vi "phan_upgrade9_12.vi"() -> ()   [LabVIEW 2019]
uses:
  <vilib>/myRIO/Instrument Drivers/Onboard IO/I2C/typedefs/I2C User Configuration.ctl
  <vilib>/myRIO/Instrument Drivers/Onboard IO/I2C/typedefs/I2C Transfer Rate.ctl
  <vilib>/Platform/TimedLoop/XDataNode/timing_clust.ctl
  <vilib>/Platform/TimedLoop/XDataNode/nitl_modes.ctl
  <vilib>/Platform/TimedLoop/XDataNode/wakeup.ctl
  <vilib>/myRIO/Instrument Drivers/Onboard IO/I2C/typedefs/I2C Reference.ctl
  <vilib>/myRIO/Common/Instrument Driver Framework/Utilities/typedefs/myRIO Generic Hardware Reference.ctl
  <vilib>/myRIO/Common/Instrument Driver Framework/Utilities/typedefs/Hardware Version Enum.ctl
  <vilib>/myRIO/Common/Instrument Driver Framework/Utilities/typedefs/myRIO v1.0 Reference.ctl
  <vilib>/myRIO/Common/Instrument Driver Framework/Utilities/typedefs/Generic FPGA Reference.ctl
  <vilib>/myRIO/Common/Instrument Driver Framework/myRIO v1.0/I2C/typedefs/I2C Channels Enum.ctl
  <vilib>/myRIO/Instrument Drivers/Onboard IO/I2C/typedefs/I2C Configuration.ctl
  <vilib>/userDefined/High Color/nirio_resource_hc.ctl
  <vilib>/myRIO/Common/Instrument Driver Framework/myRIO v1.0/I2C/vis/myRIO v1.1 Open I2C.vi
  <vilib>/myRIO/Common/Instrument Driver Framework/Utilities/vis/Validate Channels.vi
  <vilib>/myRIO/Common/Instrument Driver Framework/myRIO v1.0/I2C/vis/myRIO v1.0 Reserve I2C.vi
  <vilib>/myRIO/Common/Instrument Driver Framework/myRIO v1.0/UART/vis/myRIO v1.0 Close UART.vi
  <vilib>/myRIO/Common/Instrument Driver Framework/myRIO v1.0/I2C/vis/myRIO v1.0 Build MUX Configuration I2C.vi
  <vilib>/myRIO/Common/Instrument Driver Framework/myRIO v1.0/Resource Manager/vis/myRIO v1.0 Reserve Channel List.vi
  <vilib>/myRIO/Common/Instrument Driver Framework/myRIO v1.0/Resource Manager/vis/myRIO v1.0 Create Configuration List.vi
  <vilib>/myRIO/Common/Instrument Driver Framework/myRIO v1.0/Resource Manager/vis/myRIO v1.0 Reserve Channel.vi
  <vilib>/myRIO/Common/Instrument Driver Framework/myRIO v1.0/Resource Manager/vis/myRIO v1.0 Unreserve Channel.vi
  <vilib>/myRIO/Common/Instrument Driver Framework/myRIO v1.0/Resource Manager/vis/myRIO v1.0 Build Mutex Name.vi
  <vilib>/Utility/VariantDataType/GetNumericInfo.vi
  <vilib>/Utility/error.llb/Error Cluster From Error Code.vi
  <vilib>/myRIO/Common/Instrument Driver Framework/myRIO v1.0/myRIO v1.1 Open.vi
  <vilib>/myRIO/Common/Instrument Driver Framework/Utilities/vis/IO Manager.vi
  <vilib>/myRIO/Common/Instrument Driver Framework/Utilities/vis/Configuration Manager.vi
  <vilib>/myRIO/Common/Instrument Driver Framework/myRIO v1.0/Resource Manager/vis/myRIO v1.0 Configure IO.vi
  <vilib>/myRIO/Common/Instrument Driver Framework/myRIO v1.0/myRIO v1.0 Close.vi
  <vilib>/myRIO/Common/Instrument Driver Framework/myRIO v1.0/I2C/vis/myRIO v1.0 Configure I2C.vi
  <vilib>/myRIO/Common/Instrument Driver Framework/myRIO v1.0/I2C/vis/myRIO v1.0 Write I2C.vi
  <vilib>/myRIO/Common/Instrument Driver Framework/myRIO v1.0/I2C/vis/myRIO v1.0 Read I2C.vi
  <vilib>/myRIO/Common/Instrument Driver Framework/Utilities/vis/FPGA Ref Manager.vi
  <vilib>/myRIO/Common/Instrument Driver Framework/myRIO v1.0/myRIO v1.0 Reset FPGA.vi
  <vilib>/myRIO/Common/Instrument Driver Framework/myRIO v1.0/IRQ/vis/myRIO v1.0 IRQ Info FGV.vi
  <vilib>/myRIO/Common/Instrument Driver Framework/myRIO v1.0/IRQ/vis/myRIO v1.0 Timer IRQ Info FGV.vi
  <vilib>/myRIO/Common/Instrument Driver Framework/myRIO v1.0/IRQ/vis/myRIO v1.0 ISR Agent.vi
  <vilib>/myRIO/Instrument Drivers/Utilities/vis/Reset Index.vi
  <vilib>/myRIO/Common/Instrument Driver Framework/myRIO v1.0/Resource Manager/vis/myRIO v1.0 Block Write Resource Manager.vi
  <vilib>/platform/TimedLoop/XDataNode/XDataNode.xnode
  <vilib>/myRIO/Instrument Drivers/Onboard IO/I2C/vis/myRIO I2C Open.xnode
  <vilib>/Platform/TimedLoop/XDataNode/XDNodeRunTimeDep.lvlib
  <vilib>/ptbypt/NI_PtbyPt.lvlib
  <vilib>/myRIO/Instrument Drivers/Onboard IO/I2C/I2C.lvlib
  <vilib>/myRIO/Instrument Drivers/Utilities/Utilities.lvlib
panel:
  out "y":dbl(graph)
  out "x":dbl(graph)
  out "theta_ph":dbl
  out "offset":dbl
  out "gocphanhoi":dbl
  out "y_1":dbl
  out "x_1":dbl
  out "y_0":dbl
  out "x_0":dbl
  out "wpre":dbl
  out "yo":dbl
  out "xo":dbl
  out "phi_ph":dbl
  out "wdk":dbl
  out "phi_sp":dbl
  in  "Kiw":dbl
  in  "Kpw":dbl=3.0
  in  "Kdw":dbl
  out "Vxdk":dbl
  out "Vydk":dbl
  in  "Kdv3":dbl
  in  "Kiv3":dbl=30.0
  in  "Kpv3":dbl=0.7
  in  "Kdv2":dbl
  in  "Kiv2":dbl=30.0
  in  "Kpv2":dbl=0.7
  out "Ts":dbl=10.0
  out "sailechvitri":cluster{"e_phi":dbl, "e_x":dbl, "e_y":dbl}(graph)
  in  "Kdxy":dbl
  in  "Kixy":dbl
  in  "Kpxy":dbl=4.0
  in  "?":T1(tab)
  out "time":dbl
  in  "phi_start":dbl=1.57 format="%#_13g"
  in  "phi_end":dbl=18.85
  in  "x0":dbl
  in  "w":dbl=0.2
  in  "y0":dbl
  in  "R":dbl=1.0
  in  "R":dbl=0.6
  in  "phi_end":dbl=18.85
  in  "phi_start":dbl format="%#_13g"
  in  "x0":dbl
  in  "w":dbl=0.5
  out "time 2":dbl
  in  "y0":dbl
  out "time":dbl
  in  "x":dbl
  in  "y":dbl
  in  "CONT":bool
  in  "vantoc":dbl=0.3
  in  "x0":dbl
  in  "y0":dbl
  in  "vx":dbl
  in  "vy":dbl
  out "time":dbl
  out "time 3":dbl
  in  "phi_start 2":dbl format="%#_13g"
  in  "phi_end 2":dbl=31.4
  in  "x0 2":dbl
  in  "w 2":dbl=0.2
  in  "y0 2":dbl
  out "w_ph3":dbl
  out "w_ph2":dbl
  out "w_ph1":dbl
  in  "RESETMAP":bool=TRUE caption="Reset"
  out "duty3":dbl
  out "duty2":dbl
  out "duty1":dbl
  in  "RESET":bool
  out "Y_sp":dbl
  out "X_sp":dbl
  out "Y_ph":dbl
  out "X_ph":dbl
  out "Map":cluster{"Y":dbl[], "Y":dbl[]}[](graph)
  out "V3_sp":dbl
  out "V3_ph":dbl
  out "VAN TOC":T2(graph)
  in  "Kdv1":dbl
  in  "Kiv1":dbl=30.0
  in  "Kpv1":dbl=0.7
  out "V2_ph":dbl
  out "V1_ph":dbl
  out "V2_sp":dbl
  out "V1_sp":dbl
  in  "START":bool
  # "HE THONG"
  # "PID VI TRI"
  # "PID TOC DO"
  # "VI TRI DIEU KHIEN\n(m)"
  # "VI TRI PHAN HOI\n(m)"
  # "Van toc dat"
  # "VAN TOC DIEU KHIEN\n(m/s)"
  # "VAN TOC PHAN HOI\n(m/s)"
  # "DUTY"
  # "TOC DO PHAN HOI (rad/s)"
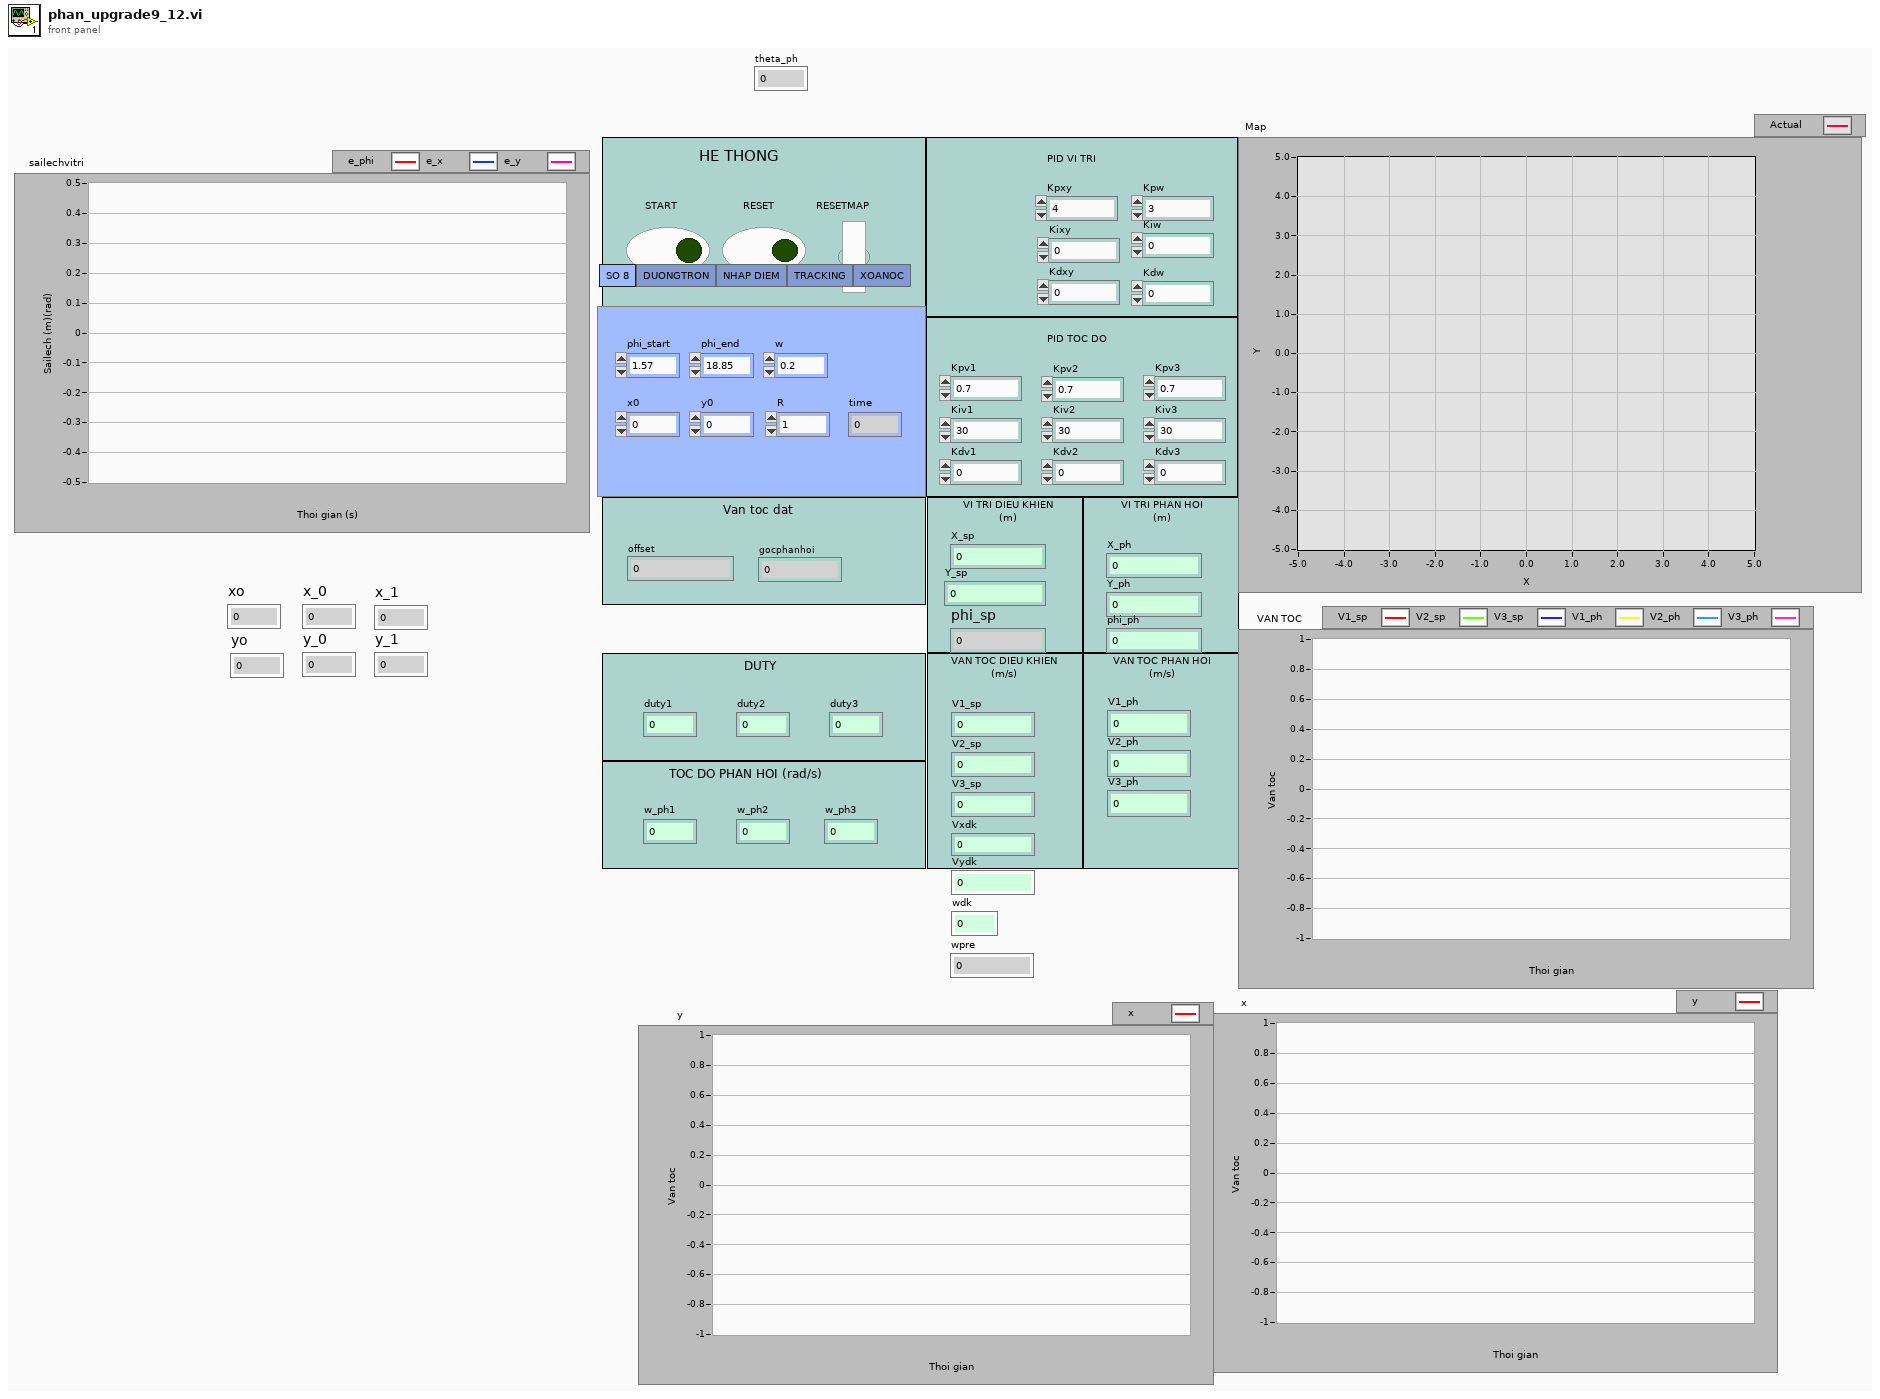
[diagram p1: front panel]
types:
  T1 = enum32{"SO 8", "DUONGTRON", "NHAP DIEM", "TRACKING", "XOANOC"}
  T2 = cluster{dbl, dbl, "V1_ph":dbl, "V2_ph":dbl, dbl, "V3_ph":dbl}
  T3 = typedef "I2C.lvlib/I2C User Configuration.ctl" = cluster{"I2C Transfer Rate":T4}
  T4 = typedef "I2C.lvlib/I2C Transfer Rate.ctl" = enum16{"Standard mode (100 kbps)", "Fast mode (400 kbps)"}
  T5 = typedef "XDNodeRunTimeDep.lvlib/timing_clust.ctl" = cluster{"Expected End [f-1]":u64, "Actual End [f-1]":u64, "Finished Late? [f-1]":bool, "Expected End [i-1]":u64, "Actual End [i-1]":u64, "Finished Late? [i-1]":bool, "Expected Start [i]":u64, "Actual Start [i]":u64, "Expected Start [f]":u64, "Actual Start [f]":u64, "Source Name":string, "Structure Name":string, "Period":i64, "Deadline":i64, "Offset":i64, "Start":i64, "Priority":i32, "Timeout":i32, "Mode":T6, "Wakeup Reason":T7, "Error":errorcluster, "Source Type":string, "Secondary Source Type":string, "Global End Time":u64, "Global Start Time":u64, "Frame Duration":u64, "Iteration Duration":u64, "Assigned CPU":i32, "I/O Scan Engine Mode":u32}
  T6 = typedef "XDNodeRunTimeDep.lvlib/nitl_modes.ctl" = enum32{"No Change", "Process missed periods, maintain original phase", "Discard missed periods, maintain original phase", "Process missed periods, ignore original phase", "Discard missed periods, ignore original phase"}
  T7 = typedef "XDNodeRunTimeDep.lvlib/wakeup.ctl" = enum32{"Normal", "Aborted", "Asynchronous wakeup", "Timing source error", "Timed loop error", "Timeout"}
  T8 = typedef "I2C.lvlib/I2C Reference.ctl" = cluster{"myRIO Reference":T9, "I2C Channels Enum":T13, "I2C Configuration":T14}
  T9 = typedef "myRIO Generic Hardware Reference.ctl" = cluster{"myRIO Model":T10, "myRIO Hardware Reference":T11}
  T10 = typedef "Hardware Version Enum.ctl" = enum16{"Unknown", "myRIO-1900", "myRIO-1950", "roboRIO", "NI ELVIS RIO CM", "ELVIS III"}
  T11 = typedef "myRIO v1.0 Reference.ctl" = cluster{"Generic FPGA Reference":T12, "Allow multiple opens":bool}
  T12 = typedef "Generic FPGA Reference.ctl" = refnum<k20>
  T13 = typedef "I2C Channels Enum.ctl" = enum16{"Not Connected", "A/I2C", "B/I2C", "I2C/I2C"}
  T14 = typedef "I2C.lvlib/I2C Configuration.ctl" = cluster{"I2C Transfer Rate":T4}
  T15 = cluster{"V1_sp":dbl, "V2_sp":dbl, "V3_sp":dbl, "V_ph1":dbl, "V_ph2":dbl, "V_ph3":dbl}
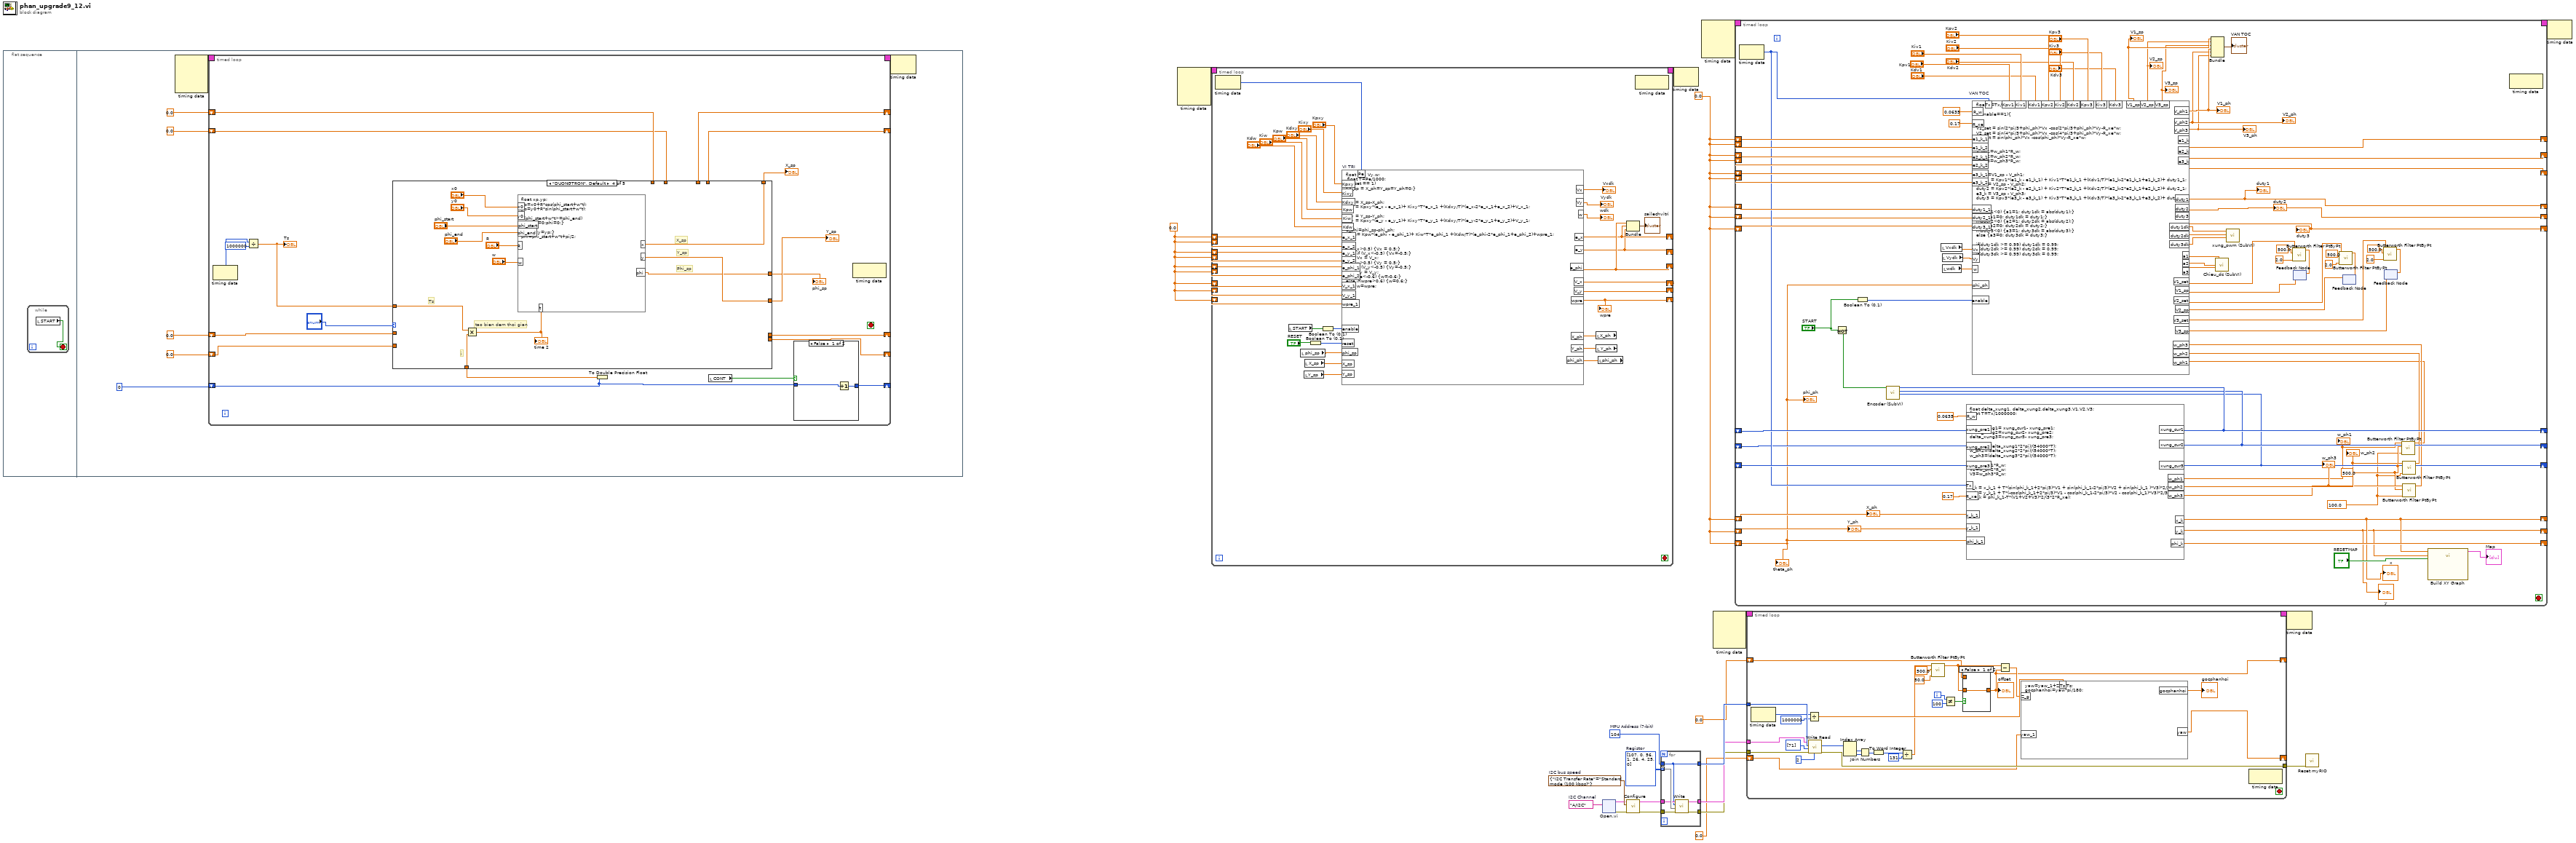
[diagram p0: block diagram]
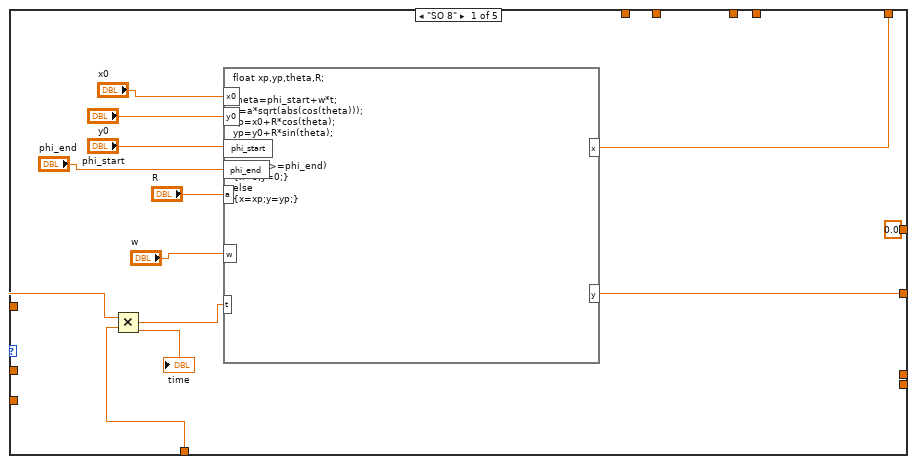
[diagram p3: hidden frame]
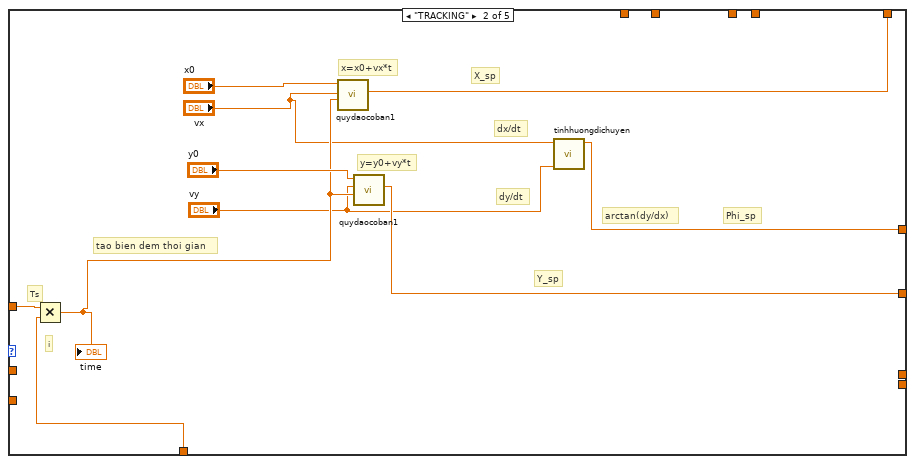
[diagram p4: hidden frame]
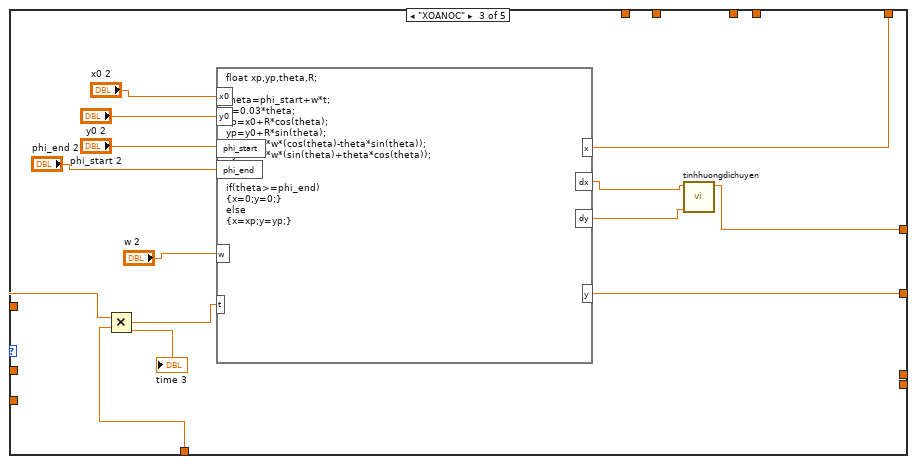
[diagram p5: hidden frame]
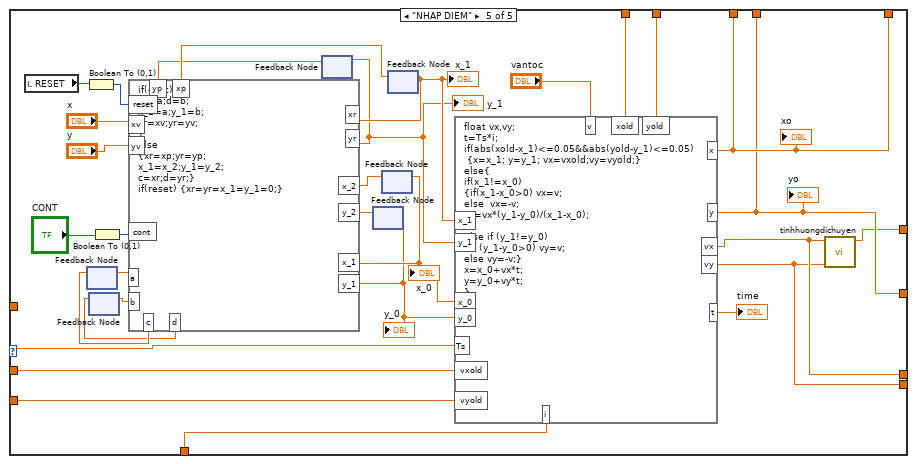
[diagram p6: hidden frame]
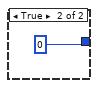
[diagram p7: hidden frame]
diagram:
  w9 = u8[][] [[107, 0], [56, 1], [26, 4], [25, 0]]  # Registor
  w8 = u8 104  # MPU Address (7-bit)
  w13 = T3 {"I2C Transfer Rate"=enum."Standard mode (100 kbps)"}  # I2C bus speed
  w14 = tag "A/I2C"  # I2C Channel
  w17 = 0.0 ("e_x")
  w18 = 0.0 ("e1")
  n1 = flat-sequence {
    frame #0 {
      n2 = while {
        stop <- w23 stop-if-true
        n3 = local read "START"() -> (w23:bool)
      }
    }
    frame #1 {
      n4 = node-c288() -> (w30:T5)  [unwired: 4 in]
      n5 = timed-loop {
        timing: w30 -> [_]
        timing-out: [_] -> w29
        shift-right: [w48] -> _
        shift-left: 0 -> [w47]
        shift-right: [w38] -> _
        shift-left: 0.0 -> [w36]
        shift-right: [w37] -> _
        shift-left: 0.0 -> [w35]
        shift-right: [w34] -> _
        shift-left: 0.0 ("x") -> [w32]
        shift-right: [w33] -> _
        shift-left: 0.0 ("y") -> [w31]
        stop <- _ stop-if-true
        n6 = node-c288() -> (w46:i64)  [unwired: 1 in]
        n7 = Divide(x=w46, y=i64 1000000) -> (x/y=w43:dbl)
        "Ts" <- w43
        n8 = To Double Precision Float(number=w47) -> (double precision float=w49:dbl)
        n9 = case shown="\"DUONGTRON\", Default" "?" {
          tunnel: w49 -> [w60 w71 w77 w95 w127]
          tunnel: [w52 w68 w75 w87 w101] -> w42
          tunnel: [w51 w65 w76 w86 w100] -> w41
          tunnel: [0.0 ("phi_0") w62 w72 w85 w97] -> w40
          tunnel: w43 -> [w61 w70 w78 w96 w107]
          tunnel: [_ _ _ _ w105] -> w38
          tunnel: [_ _ _ _ w104] -> w37
          tunnel: w36 -> [_ _ _ _ w103]
          tunnel: w35 -> [_ _ _ _ w102]
          tunnel: [_ _ _ _ w101] -> w34
          tunnel: [_ _ _ _ w100] -> w33
          tunnel: w32 -> [_ _ _ _ w99]
          tunnel: w31 -> [_ _ _ _ w98]
          frame "SO 8" {
            n10 = Multiply(x=w61, y=w60) -> (x*y=w59:dbl)
            "time" <- w59
            n11 = formula code="float xp,yp,theta,R;\n\ntheta=phi_start+w*t;\nR=a*sqrt(abs(cos(theta)));\nxp=x0+R*cos(theta);\nyp=y0+R*sin(theta);\n\n\nif(theta>=phi_end)\n{x=0;y=0;}\nelse\n{x=xp;y=yp;}"("t"=w59, "w"="w", "x0"="x0", "y0"="y0", "phi_start"="phi_start", "phi_end"="phi_end", "a"="R") -> ("x"=w52:dbl, "y"=w51:dbl)
          }
          frame "TRACKING" {
            # "Y_sp"
            # "Phi_sp"
            # "X_sp"
            # "arctan(dy/dx)"
            # "dy/dt"
            # "dx/dt"
            # "Ts"
            # "i"
            # "y=y0+vy*t"
            # "x=x0+vx*t"
            # "tao bien dem thoi gian"
            n12 = Multiply(x=w70, y=w71) -> (x*y=w66:dbl)
            "time" <- w66
            n13 = call "quydaocoban1.vi"("t"=w66, "v"="vx", "S0"="x0") -> ("S"=w68:dbl)  [unwired: 8 in]
            n14 = call "quydaocoban1.vi"("t"=w66, "v"="vy", "S0"="y0") -> ("S"=w65:dbl)  [unwired: 8 in]
            n15 = call "tinhhuongdichuyen.vi"("dy"="vy", "dx"="vx") -> ("phi"=w62:dbl)  [unwired: 9 in]
          }
          frame "XOANOC" {
            n16 = Multiply(x=w78, y=w77) -> (x*y=w84:dbl)
            "time 3" <- w84
            n17 = formula code="float xp,yp,theta,R;\n\ntheta=phi_start+w*t;\nR=0.03*theta;\nxp=x0+R*cos(theta);\nyp=y0+R*sin(theta);\ndx=0.03*w*(cos(theta)-theta*sin(theta));\ndy=0.03*w*(sin(theta)+theta*cos(theta));\n\n\nif(theta>=phi_end)\n{x=0;y=0;}\nelse\n{x=xp;y=yp;}"("t"=w84, "w"="w 2", "x0"="x0 2", "y0"="y0 2", "phi_start"="phi_start 2", "phi_end"="phi_end 2") -> ("x"=w75:dbl, "y"=w76:dbl, "dx"=w74:dbl, "dy"=w73:dbl)
            n18 = call "tinhhuongdichuyen.vi"("dy"=w73, "dx"=w74) -> ("phi"=w72:dbl)  [unwired: 9 in]
          }
          frame "DUONGTRON", Default {
            # "Phi_sp"
            # "Y_sp"
            # "X_sp"
            # "i"
            # "Ts"
            # "tao bien dem thoi gian"
            n19 = Multiply(x=w96, y=w95) -> (x*y=w94:dbl)
            "time 2" <- w94
            n20 = formula code="float xp,yp;\nxp=x0+R*cos(phi_start+w*t);\nyp=y0+R*sin(phi_start+w*t);\n\nif(phi_start+w*t>=phi_end)\n{x=0;y=0;phi=0;}\nelse\n{x=xp;y=yp;}\nphi=phi_start+w*t+pi/2;"("t"=w94, "w"="w", "x0"="x0", "y0"="y0", "phi_start"="phi_start", "phi_end"="phi_end", "R"="R") -> ("x"=w87:dbl, "y"=w86:dbl, "phi"=w85:dbl)
          }
          frame "NHAP DIEM" {
            n21 = local read "RESET"() -> (w109:bool)
            n22 = Boolean To (0,1)(Boolean=w109) -> (0, 1=w108:i16)
            n23 = feedback #1() -> (w112:dbl)  [unwired: 1 in]
            n24 = feedback #2() -> (w110:dbl)  [unwired: 1 in]
            n25 = Boolean To (0,1)(Boolean="CONT") -> (0, 1=w124:i16)
            n26 = feedback #3() -> (w118:dbl)  [unwired: 1 in]
            n27 = feedback #4() -> (w115:dbl)  [unwired: 1 in]
            n28 = feedback #5() -> (w117:dbl)  [unwired: 1 in]
            n29 = feedback #6() -> (w119:dbl)  [unwired: 1 in]
            n30 = formula code="if(cont)\n{c=a;d=b;\nx_1=a;y_1=b;\nxr=xv;yr=yv;\n}\nelse \n{xr=xp;yr=yp;\nx_1=x_2;y_1=y_2;\nc=xr;d=yr;}\nif(reset) {xr=yr=x_1=y_1=0;}"("cont"=w124, "xv"="x", "yv"="y", "yp"=w118, "xp"=w119, "x_2"=w117, "y_2"=w115, "a"=w112, "b"=w110, "reset"=w108) -> ("xr"=w121:dbl, "yr"=w120:dbl, "x_1"=w116:dbl, "y_1"=w114:dbl, "c"=w113:dbl, "d"=w111:dbl)
            "x_0" <- w116
            "y_0" <- w114
            "x_1" <- w121
            "y_1" <- w120
            n31 = feedback-in #1(w113) -> ()
            n32 = feedback-in #2(w111) -> ()
            n33 = feedback-in #3(w120) -> ()
            n34 = feedback-in #4(w114) -> ()
            n35 = feedback-in #5(w116) -> ()
            n36 = feedback-in #6(w121) -> ()
            n37 = formula code="float vx,vy;\nt=Ts*i;\nif(abs(xold-x_1)<=0.05&&abs(yold-y_1)<=0.05)\n {x=x_1; y=y_1; vx=vxold;vy=vyold;}\nelse{\nif(x_1!=x_0)\n{if(x_1-x_0>0) vx=v;\nelse  vx=-v;\nvy=vx*(y_1-y_0)/(x_1-x_0);\n}\nelse if (y_1!=y_0) \n{if (y_1-y_0>0) vy=v;\nelse vy=-v;}\nx=x_0+vx*t;\ny=y_0+vy*t;\n}"("i"=w127, "x_1"=w121, "y_1"=w120, "x_0"=w116, "y_0"=w114, "Ts"=w107, "v"="vantoc", "xold"=w99, "yold"=w98, "vxold"=w103, "vyold"=w102) -> ("x"=w101:dbl, "y"=w100:dbl, "vx"=w105:dbl, "t"=→"time":dbl, "vy"=w104:dbl)
            "xo" <- w101
            "yo" <- w100
            n38 = call "tinhhuongdichuyen.vi"("dy"=w104, "dx"=w105) -> ("phi"=w97:dbl)  [unwired: 9 in]
          }
        }
        "X_sp" <- w42
        "Y_sp" <- w41
        "phi_sp" <- w40
        n39 = local read "CONT"() -> (w44:bool)
        n40 = case shown="False" w44 {
          tunnel: [w129 0] -> w48
          tunnel: w47 -> [w128 _]
          frame False {
            n41 = Increment(x=w128) -> (x+1=w129:i32)
          }
          frame True {
          }
        }
        n42 = node-c288() -> ()  [unwired: 1 in, 1 out]
      }
      n43 = node-c288(w29) -> ()  [unwired: 1 out]
    }
  }
  n44 = node-c288() -> (w20:T5)  [unwired: 4 in]
  n45 = timed-loop {
    timing: w20 -> [_]
    timing-out: [_] -> w19
    shift-right: [w156] -> _
    shift-left: w17 -> [w164]
    shift-left: w17 -> [w163]
    shift-right: [w142] -> _
    shift-left: w17 -> [w162]
    shift-left: w17 -> [w161]
    shift-right: [w157] -> _
    shift-left: w17 -> [w160]
    shift-left: w17 -> [w159]
    shift-right: [w147] -> _
    shift-left: w17 -> [w150]
    shift-right: [w146] -> _
    shift-left: w17 -> [w149]
    shift-right: [w145] -> _
    shift-left: w17 -> [w148]
    stop <- _ stop-if-true
    # "Gioihantocdo"
    # "BodieukhienPIDvitri"
    n46 = node-c288() -> (w171:i64)  [unwired: 1 in]
    n47 = local read "START"() -> (w144:bool)
    n48 = local read "phi_sp"() -> (w140:dbl)
    n49 = local read "Y_sp"() -> (w139:dbl)
    n50 = local read "X_sp"() -> (w141:dbl)
    n51 = Boolean To (0,1)(Boolean="RESET") -> (0, 1=w154:i16)
    n52 = Boolean To (0,1)(Boolean=w144) -> (0, 1=w143:i16)
    n53 = local read "X_ph"() -> (w153:dbl)
    n54 = local read "Y_ph"() -> (w152:dbl)
    n55 = local read "phi_ph"() -> (w151:dbl)
    n56 = formula code="float  Vx, Vy,w;\n float T=Pe/1000;\nif(reset == 1)\n{X_sp = X_ph=Y_sp=Y_ph=0;}\n \n\ne_x = X_sp-X_ph; \nV_x = Kpxy*(e_x - e_x_1)+ Kixy*T*e_x_1 +(Kdxy/T)*(e_x-2*e_x_1+e_x_2)+V_x_1;\n\ne_y = Y_sp-Y_ph; \nV_y = Kpxy*(e_y - e_y_1)+ Kixy*T*e_y_1 +(Kdxy/T)*(e_y-2*e_y_1+e_y_2)+V_y_1;\n\ne_phi=phi_sp-phi_ph;\nwpre= Kpw*(e_phi - e_phi_1)+ Kiw*T*e_phi_1 +(Kdw/T)*(e_phi-2*e_phi_1+e_phi_2)+wpre_1;\n\n\nif (V_x>0.5) {Vx = 0.5;} \nelse if (V_x<-0.5) {Vx=-0.5;}\nelse Vx = V_x;\nif (V_y>0.5) {Vy = 0.5;} \nelse if (V_y<-0.5) {Vy=-0.5;}\nelse Vy = V_y;\nif (wpre<-0.6) {w=-0.6;}\nelse if(wpre>0.6) {w=0.6;}\nelse w=wpre;" "VI TRI"("Kpxy"="Kpxy", "Kixy"="Kixy", "Kdxy"="Kdxy", "Kpw"="Kpw", "Kiw"="Kiw", "Kdw"="Kdw", "Pe"=w171, "e_x_1"=w164, "e_x_2"=w163, "e_y_1"=w162, "e_y_2"=w161, "e_phi_1"=w160, "e_phi_2"=w159, "reset"=w154, "phi_sp"=w140, "X_sp"=w141, "Y_sp"=w139, "X_ph"=w153, "Y_ph"=w152, "phi_ph"=w151, "V_x_1"=w150, "V_y_1"=w149, "wpre_1"=w148, "enable"=w143) -> ("e_x"=w156:dbl, "e_y"=w142:dbl, "e_phi"=w157:dbl, "Vx"=→"Vxdk":dbl, "Vy"=→"Vydk":dbl, "w"=→"wdk":dbl, "V_x"=w147:dbl, "V_y"=w146:dbl, "wpre"=w145:dbl)
    "wpre" <- w145
    n57 = Bundle("e_phi"=w157, "e_x"=w156, "e_y"=w142) -> (→"sailechvitri":cluster{"e_phi":dbl, "e_x":dbl, "e_y":dbl})  [unwired: 1 in]
    n58 = node-c288() -> ()  [unwired: 1 in, 1 out]
  }
  n59 = xnode "Open.vi"("Channel Name"=w14) -> ("error out"=w11:errorcluster, "I2C Ref Out"=w12:T8)  [unwired: 2 in]
  n60 = call <vilib>:"Configure.vi"("error in (no error)"=w11, "I2C User Configuration"=w13, "I2C Ref In"=w12) -> ("error out"=w10:errorcluster, "I2C Ref Out"=w6:T8)  [unwired: 7 in]
  n61 = for {
    tunnel: w10 -> [w180]
    tunnel: w8 -> [w177]
    tunnel: w9 -> [w179] mode=indexing
    tunnel: w6 -> [w178]
    tunnel: [w177] -> w5
    tunnel: [w176] -> w4
    tunnel: [w175] -> w3
    n62 = call <vilib>:"Write.vi"("error in (no error)"=w180, "Bytes to Write"=w179, "Slave Address (7-bit)"=w177, "I2C Ref In"=w178) -> ("error out"=w175:errorcluster, "I2C Ref Out"=w176:T8)  [unwired: 6 in]
  }
  n63 = node-c288(w19) -> ()  [unwired: 1 out]
  n64 = node-c288() -> (w22:T5)  [unwired: 4 in]
  n65 = node-c288() -> (w16:T5)  [unwired: 4 in]
  n66 = timed-loop {
    timing: w22 -> [_]
    timing-out: [_] -> w21
    shift-right: [w265] -> _
    shift-left: w18 -> [w263]
    shift-right: [w264] -> _
    shift-left: w18 -> [w242]
    shift-right: [w257] -> _
    shift-left: w18 -> [w256]
    shift-right: [w182] -> _
    shift-left: w18 -> [w200]
    shift-right: [w181] -> _
    shift-left: w18 -> [w199]
    shift-right: [w253] -> _
    shift-left: w18 -> [w251]
    shift-right: [w252] -> _
    shift-left: w18 -> [w201]
    shift-right: [w207] -> _
    shift-left: w18 -> [w250]
    shift-right: [w245] -> _
    shift-left: _ -> [w247]
    shift-right: [w244] -> _
    shift-left: _ -> [w206]
    shift-right: [w243] -> _
    shift-left: _ -> [w246]
    shift-left: w18 -> [w241]
    shift-left: w18 -> [w240]
    shift-left: w18 -> [w239]
    shift-right: [w205] -> _
    shift-left: w18 -> [w190]
    stop <- _ stop-if-true
    w235 = 100.0 ("flw")
    w236 = 500.0 ("sampling freq: fs")
    # "phat xung dieu khien va huong quay banh xe"
    # "bodieukhienvantoc"
    # "vantocphanhoi"
    # "tinh van toc 3 banh xe tu dong hoc nghich"
    # "Tinh vi tri phan hoi tu van toc qua dong hoc thuan"
    # "Tinh van toc phan hoi tu  encoder"
    n67 = node-c288() -> (w208:i64)  [unwired: 1 in]
    n68 = Not(x="START") -> (.not. x?=w254:bool)
    n69 = Boolean To (0,1)(Boolean="START") -> (0, 1=w262:i16)
    n70 = call "Encoder (SubVI).vi"("Boolean"=w254) -> ("Counter Value3"=w243:i32, "Counter Value 2"=w244:i32, "Counter Value"=w245:i32)  [unwired: 8 in]
    n71 = local read "Vxdk"() -> (w198:dbl)
    n72 = local read "Vydk"() -> (w197:dbl)
    n73 = local read "wdk"() -> (w196:dbl)
    n74 = formula code="float delta_xung1, delta_xung2,delta_xung3,V1,V2,V3;\nfloat T=Tx/1000000;\n\n\ndelta_xung1= xung_cur1- xung_pre1;\ndelta_xung2=xung_cur2- xung_pre2;\ndelta_xung3=xung_cur3- xung_pre3; \n\nw_ph1=(delta_xung1*2*pi)/(54000*T);\nw_ph2=(delta_xung2*2*pi)/(54000*T);\nw_ph3=(delta_xung3*2*pi)/(54000*T);\n\nV1=w_ph1*R_w;\nV2=w_ph2*R_w;\nV3=w_ph3*R_w;\n\n\nx_k = x_k_1 + T*(sin(phi_k_1+2*pi/3)*V1 + sin(phi_k_1-2*pi/3)*V2 + sin(phi_k_1 )*V3)*2/3;\ny_k = y_k_1 + T*(-cos(phi_k_1+2*pi/3)*V1 - cos(phi_k_1-2*pi/3)*V2 - cos(phi_k_1)*V3)*2/3;\nphi_k = phi_k_1-T*(V1+V2+V3)*2/(3*2*R_xe);"("xung_pre1"=w247, "xung_pre2"=w206, "xung_pre3"=w246, "xung_cur1"=w245, "xung_cur2"=w244, "xung_cur3"=w243, "Tx"=w208, "x_k_1"=w200, "y_k_1"=w199, "phi_k_1"=w190, "R_w"=0.0635 ("input variable"), "R_xe"=0.17 ("input variable")) -> ("w_ph1"=w226:dbl, "w_ph2"=w238:dbl, "w_ph3"=w237:dbl, "x_k"=w182:dbl, "y_k"=w181:dbl, "phi_k"=w205:dbl)
    "w_ph1" <- w226
    "w_ph2" <- w238
    "w_ph3" <- w237
    "x" <- w182
    "y" <- w181
    n75 = feedback #7() -> (w216:dbl)  [unwired: 1 in]
    n76 = feedback #8() -> (w213:dbl)  [unwired: 1 in]
    n77 = feedback #9() -> (w210:dbl)  [unwired: 1 in]
    n78 = call <vilib>:"Butterworth Filter PtByPt.vi"("low cutoff freq: fl"=w235, "sampling freq: fs"=w236, "x"=w226) -> ("Filtered x"=w225:dbl)  [unwired: 6 in, 1 out]
    n79 = call <vilib>:"Butterworth Filter PtByPt.vi"("low cutoff freq: fl"=w235, "sampling freq: fs"=w236, "x"=w238) -> ("Filtered x"=w234:dbl)  [unwired: 6 in, 1 out]
    n80 = call <vilib>:"Butterworth Filter PtByPt.vi"("low cutoff freq: fl"=w235, "sampling freq: fs"=w236, "x"=w237) -> ("Filtered x"=w233:dbl)  [unwired: 6 in, 1 out]
    n81 = formula code="float T=Tx/1000000;\n\nif(enable==1){\n\n\nV1_set = sin(2*pi/3+phi_ph)*Vx -cos(2*pi/3+phi_ph)*Vy-R_xe*w;\nV2_set = sin(4*pi/3+phi_ph)*Vx -cos(4*pi/3+phi_ph)*Vy-R_xe*w;\nV3_set = sin(phi_ph)*Vx -cos(phi_ph)*Vy-R_xe*w;\n\n\nV_ph1=w_ph1*R_w;\nV_ph2=w_ph2*R_w;\nV_ph3=w_ph3*R_w;\n\n\ne1_k =V1_sp - V_ph1;\nduty1 = Kpv1*(e1_k - e1_k_1) + Kiv1*T*e1_k_1 +(Kdv1/T)*(e1_k-2*e1_k_1+e1_k_2)+ duty1_1;\ne2_k = V2_sp - V_ph2;\nduty2 = Kpv2*(e2_k - e2_k_1) + Kiv2*T*e2_k_1 +(Kdv2/T)*(e2_k-2*e2_k_1+e2_k_2)+ duty2_1;\ne3_k = V3_sp - V_ph3;\nduty3 = Kpv3*(e3_k - e3_k_1) + Kiv3*T*e3_k_1 +(Kdv3/T)*(e3_k-2*e3_k_1+e3_k_2)+ duty3_1;\n\n\nif(duty1<0) {a1=1; duty1dk = abs(duty1);}\nelse {a1=0; duty1dk = duty1;}\nif(duty2<0) {a2=1; duty2dk = abs(duty2);}\nelse {a2=0; duty2dk = duty2;}\nif(duty3<0) {a3=1; duty3dk = abs(duty3);}\nelse {a3=0; duty3dk = duty3;}\n\nif(duty1dk >= 0.99) duty1dk = 0.99;\nif(duty2dk >= 0.99) duty2dk = 0.99;\nif(duty3dk >= 0.99) duty3dk = 0.99;\n}" "VAN TOC"("Kpv1"="Kpv1", "Kiv1"="Kiv1", "Kdv1"="Kdv1", "e1_k_1"=w263, "e2_k_1"=w242, "enable"=w262, "Tx"=w208, "e3_k_1"=w256, "duty1_1"=w251, "duty2_1"=w201, "duty3_1"=w250, "w_ph1"=w225, "w_ph2"=w234, "w_ph3"=w233, "e1_k_2"=w241, "e2_k_2"=w240, "e3_k_2"=w239, "Kpv2"="Kpv2", "Kiv2"="Kiv2", "Kdv2"="Kdv2", "Kpv3"="Kpv3", "Kiv3"="Kiv3", "Kdv3"="Kdv3", "V1_sp"=w216, "V2_sp"=w213, "V3_sp"=w210, "R_w"=0.0635 ("input variable"), "R_xe"=0.17 ("input variable"), "Vx"=w198, "Vy"=w197, "w"=w196, "phi_ph"=w190) -> ("V1_sp"=w189:dbl, "V_ph1"=w186:dbl, "V_ph2"=w185:dbl, "e1_k"=w265:dbl, "e2_k"=w264:dbl, "V2_sp"=w188:dbl, "duty1"=w253:dbl, "duty2"=w252:dbl, "e3_k"=w257:dbl, "V_ph3"=w184:dbl, "V3_sp"=w187:dbl, "duty3"=w207:dbl, "a1"=w194:dbl, "a2"=w249:dbl, "a3"=w248:dbl, "duty1dk"=w192:dbl, "duty2dk"=w191:dbl, "duty3dk"=w193:dbl, "V1_set"=w218:dbl, "V2_set"=w215:dbl, "V3_set"=w212:dbl)
    "V1_sp" <- w189
    "V2_sp" <- w188
    "V1_ph" <- w186
    "V2_ph" <- w185
    "V3_ph" <- w184
    "V3_sp" <- w187
    "duty1" <- w253
    "duty2" <- w252
    "duty3" <- w207
    n82 = Bundle("V1_sp"=w189, "V2_sp"=w188, "V3_sp"=w187, "V_ph1"=w186, "V_ph2"=w185, "V_ph3"=w184) -> (→"VAN TOC":T15)  [unwired: 1 in]
    n83 = call "Chieu_dc (SubVI).vi"("a3"=w248, "a2"=w249, "a1"=w194) -> ()
    n84 = call "xung_pwm (SubVI).vi"("duty3 in"=w193, "duty2 in"=w191, "duty1 in"=w192) -> ()  [unwired: 6 in, 3 out]
    n85 = call <vilib>:"Butterworth Filter PtByPt.vi"("low cutoff freq: fl"=2.0, "sampling freq: fs"=500.0, "x"=w218) -> ("Filtered x"=w217:dbl)  [unwired: 6 in, 1 out]
    n86 = feedback-in #7(w217) -> ()
    n87 = call <vilib>:"Butterworth Filter PtByPt.vi"("low cutoff freq: fl"=2.0, "sampling freq: fs"=500.0, "x"=w215) -> ("Filtered x"=w214:dbl)  [unwired: 6 in, 1 out]
    n88 = feedback-in #8(w214) -> ()
    n89 = call <vilib>:"Butterworth Filter PtByPt.vi"("low cutoff freq: fl"=2.0, "sampling freq: fs"=500.0, "x"=w212) -> ("Filtered x"=w211:dbl)  [unwired: 6 in, 1 out]
    n90 = feedback-in #9(w211) -> ()
    n91 = call "Build XY Graph"("Reset"="RESETMAP", "Y Input"=w181, "X Input"=w182) -> ("XY Graph"=→"Map":cluster{"X":dbl[], "Y":dbl[]}[])  [unwired: 7 in, 1 out]
    n92 = node-c288() -> ()  [unwired: 1 in, 1 out]
    "X_ph" <- w200
    "Y_ph" <- w199
    "phi_ph" <- w190
    "theta_ph" <- w190
  }
  n93 = timed-loop {
    timing: w16 -> [_]
    timing-out: [_] -> w15
    tunnel: [w294] -> w7
    tunnel: w5 -> [w293]
    tunnel: w4 -> [w292]
    tunnel: w3 -> [w291]
    shift-right: [w276] -> _
    shift-left: 0.0 ("yaw") -> [w281]
    shift-right: [w270] -> _
    shift-left: 0.0 ("Filtered x") -> [w274]
    i -> [w273]
    stop <- _ stop-if-true
    n94 = node-c288() -> (w288:i64)  [unwired: 1 in]
    n95 = Divide(x=w288, y=i64 1000000) -> (x/y=w282:dbl)
    n96 = call <vilib>:"Write Read.vi"("Byte Count"=u32 2, "error in (no error)"=w291, "Bytes to Write"=u8[] [71], "Slave Address (7-bit)"=w293, "I2C Ref In"=w292) -> ("error out"=w294:errorcluster, "Bytes Read"=w290:u8[])  [unwired: 3 in, 1 out]
    n97 = Index Array(array=w290) -> (element #1=w284:u8, element #2=w283:u8)  [unwired: 2 in]
    n98 = Join Numbers(hi=w284, lo=w283) -> ((hi.lo)=w289:u16)
    n99 = To Word Integer(number=w289) -> (16bit integer=w286:i16)
    n100 = Divide(x=w286, y=i16 131) -> (x/y=w280:dbl)
    n101 = call <vilib>:"Butterworth Filter PtByPt.vi"("low cutoff freq: fl"=50.0, "sampling freq: fs"=500.0, "x"=w280) -> ("Filtered x"=w275:dbl)  [unwired: 6 in, 1 out]
    n102 = Not Equal?(x=w273, y=100) -> (x != y?=w271:bool)
    n103 = case shown="False" w271 {
      tunnel: w275 -> [w297 _]
      tunnel: [w297 w298] -> w270
      tunnel: w274 -> [_ w298]
      frame False {
      }
      frame True {
      }
    }
    "offset" <- w270
    n104 = Subtract(x=w275, y=w270) -> (x-y=w277:dbl)
    n105 = formula code="yaw=yaw_1+Z_g*Ts;\ngocphanhoi=yaw*pi/180;"("Z_g"=w277, "Ts"=w282, "yaw_1"=w281) -> ("yaw"=w276:dbl, "gocphanhoi"=→"gocphanhoi":dbl)
    n106 = node-c288() -> ()  [unwired: 1 in, 1 out]
  }
  n107 = node-c288(w15) -> ()  [unwired: 1 out]
  n108 = call <vilib>:"Reset myRIO.vi"("error in (no error)"=w7) -> ()  [unwired: 10 in, 1 out]
  n109 = node-c288(w21) -> ()  [unwired: 1 out]
